vi "Write array size.vi"(8 "error in (no error)":errorcluster, 10 "array size":i32, 11 "Read Multi-Point [MP] Msg in":refnum<class "Read Multi-Point [MP] Msg.lvclass">) -> (0 "error out":errorcluster, 3 "Read Multi-Point [MP] Msg out":refnum<class "Read Multi-Point [MP] Msg.lvclass">)   [LabVIEW 2015, in "CS++DMM.lvlib" / "Read Multi-Point [MP] Msg.lvclass"]
uses:
  Read Multi-Point [MP] Msg.lvclass
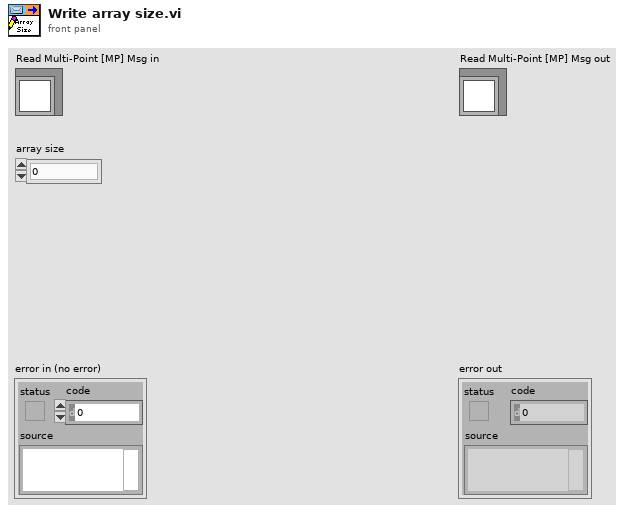
[diagram p1: front panel]
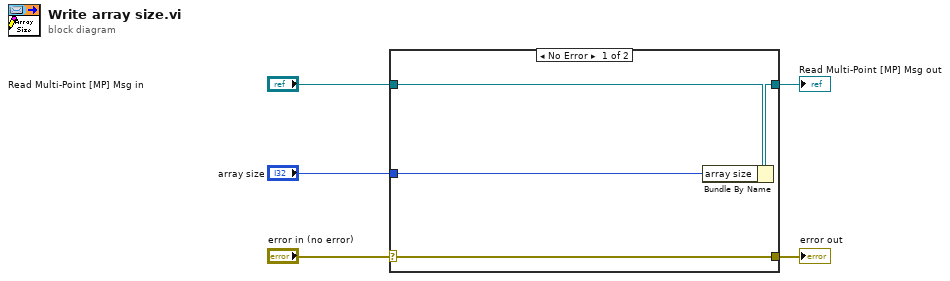
[diagram p0: block diagram]
diagram:
  n1 = case shown="No Error" "error in (no error)" {
    selector: "error in (no error)" -> [w9 w10]
    tunnel: [w9 w10] -> w4
    tunnel: [w7 w11] -> w2
    tunnel: "Read Multi-Point [MP] Msg in" -> [w8 w11]
    tunnel: "array size" -> [w6 _]
    frame No Error {
      n2 = Bundle By Name(cluster=w8, "array size"=w6) -> (w7:refnum<class "Read Multi-Point [MP] Msg.lvclass">)
    }
    frame Error {
    }
  }
  "error out" <- w4
  "Read Multi-Point [MP] Msg out" <- w2
